vi "AuMT8852B Power Control Extended Results Query.vi"(7 "Stage":T1(ring), 8 "error in (no error)":errorcluster, 11 "VISA session":refnum<visa-resource-name>) -> (0 "error out":errorcluster, 2 "error code":i32, 3 "VISA session out":refnum<visa-resource-name>, 4 "Results":T2 {"Minimum step size" format="%.2f"; "Maximum step size" format="%.2f"; "Minimum power" format="%.2f"; "Maximum power" format="%.2f"})   [LabVIEW 2017]
doc: "Anritsu MT8852B Bluetooth Tester\n\nReturns the results of the Power Control test.\n\nINPUTS\nStage - results of the individual hopping stages of the test.\n\nOUTPUTS\nResults - measurements made during the test."
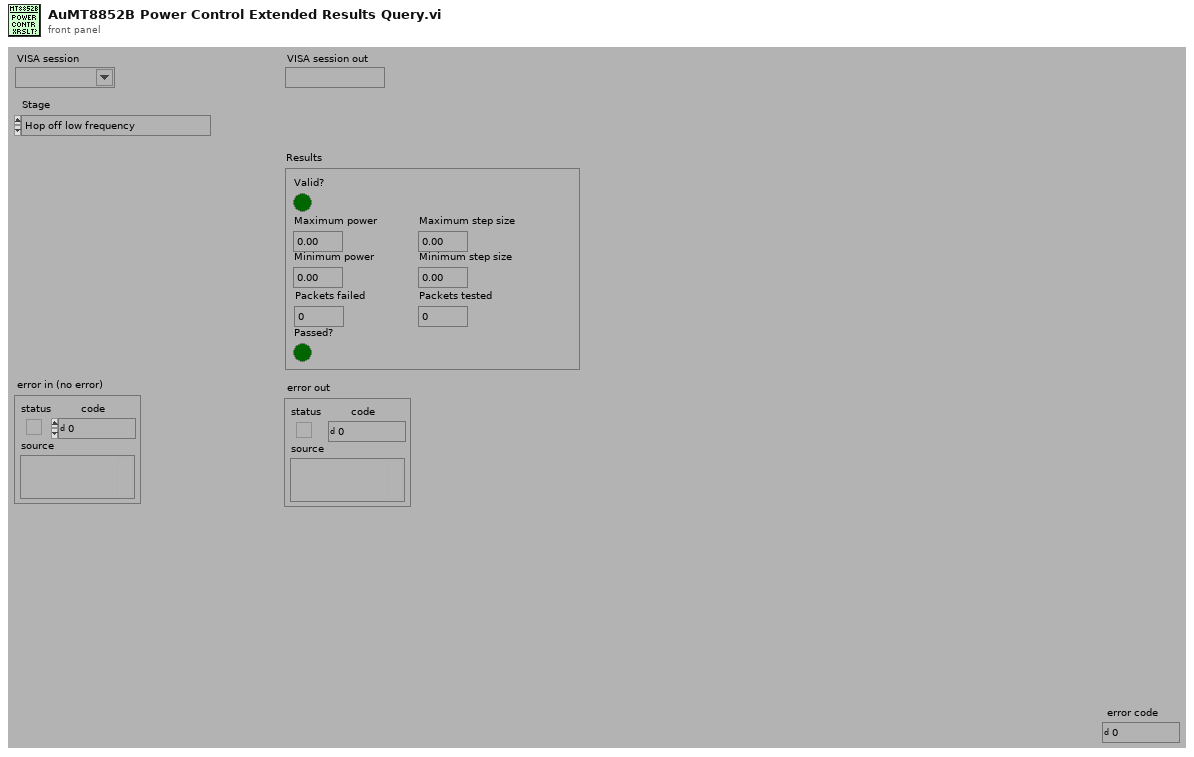
[diagram p1: front panel]
types:
  T1 = enum16{"Hop off low frequency", "Hop off medium frequency", "Hop off high frequency"}
  T2 = cluster{"Maximum power":dbl, "Minimum power":dbl, "Maximum step size":dbl, "Passed?":bool, "Minimum step size":dbl, "Valid?":bool, "Packets failed":i32, "Packets tested":i32}
  T3 = enum16{"Simulate", "Range check", "Cache", "Query instrument status"}
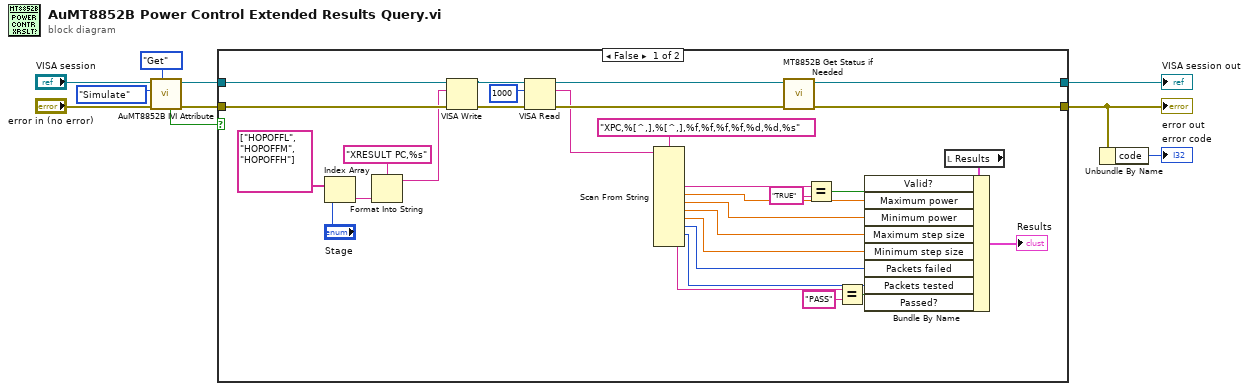
[diagram p0: block diagram]
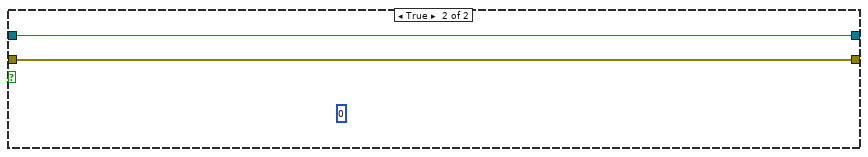
[diagram p2: hidden frame]
diagram:
  n1 = call <instrlib>:"AuMT8852B IVI Attribute.vi"("Set/Get (Set)"=enum16{"Set", "Get"}."Get", "error in (no error)"="error in (no error)", "Flag (Simulate)"=T3."Simulate", "VISA session"="VISA session") -> ("error out"=w7:errorcluster, "VISA session out"=w9:refnum<visa-resource-name>, "Value out"=w3:bool)  [unwired: 5 in]
  n2 = case shown="False" w3 {
    tunnel: [w29 w42] -> w10
    tunnel: [w28 w41] -> w1
    tunnel: w9 -> [w40 w42]
    tunnel: w7 -> [w39 w41]
    frame False {
      n3 = Index Array(array=string[] ["HOPOFFL", "HOPOFFM", "HOPOFFH"], index="Stage") -> (element=w23:string)
      n4 = Format Into String(format string="XRESULT PC,%s" ("write buffer (\"\")"), w23) -> (resulting string=w12:string)  [unwired: 2 in, 1 out]
      n5 = VISA Write(VISA resource name=w40, write buffer=w12, error in (no error)=w39) -> (VISA resource name out=w38:refnum<visa-resource-name>, error out=w37:errorcluster)  [unwired: 1 out]
      n6 = VISA Read(VISA resource name=w38, byte count=u32 1000 ("byte count (0)"), error in (no error)=w37) -> (VISA resource name out=w27:refnum<visa-resource-name>, read buffer=w11:string, error out=w26:errorcluster)  [unwired: 1 out]
      n7 = Scan From String(format string="XPC,%[^,],%[^,],%f,%f,%f,%f,%d,%d,%s" ("Format String"), input string=w11) -> (output 2=w21:string, output 3=w20:dbl, output 4=w19:dbl, output 5=w18:dbl, output 6=w17:dbl, output 7=w16:i32, output 8=w14:i32, output 9=w13:string)  [unwired: 12 in, 3 out]
      n8 = call <instrlib>:"MT8852B Get Status if Needed.vi"("error in (no error)"=w26, "VISA session"=w27) -> ("error out"=w28:errorcluster, "VISA session out"=w29:refnum<visa-resource-name>)  [unwired: 8 in]
      n9 = Equal?(x=w21, y="TRUE") -> (x = y?=w33:bool)
      n10 = Equal?(x=w13, y="PASS") -> (x = y?=w15:bool)
      n11 = local read "Results"() -> (w34:T2)
      n12 = Bundle By Name(cluster=w34, "Valid?"=w33, "Maximum power"=w20, "Minimum power"=w19, "Maximum step size"=w18, "Minimum step size"=w17, "Packets failed"=w16, "Packets tested"=w14, "Passed?"=w15) -> (→"Results":T2)
    }
    frame True {
      (unwired) u8 0
    }
  }
  "error out" <- w1
  "VISA session out" <- w10
  n13 = Unbundle By Name(w1) -> ("code"=→"error code":i32)
